vi "Devcon.Find Devices.vi"(8 "error in (no error)":errorcluster, 9 "State(Present(F), All(T))":bool, 10 "DeviceID":string="USB\\VID_28DE", 11 "DevconEXE":path=path "C:/Program Files (x86)/Windows Kits/10/Tools/x64/devcon") -> (0 "error out":errorcluster, 1 "StdOut":string, 2 "Device List":string[][](array[string]), 3 "Device Cnt":i32, 5 "Cmd":string)   [LabVIEW 2018]
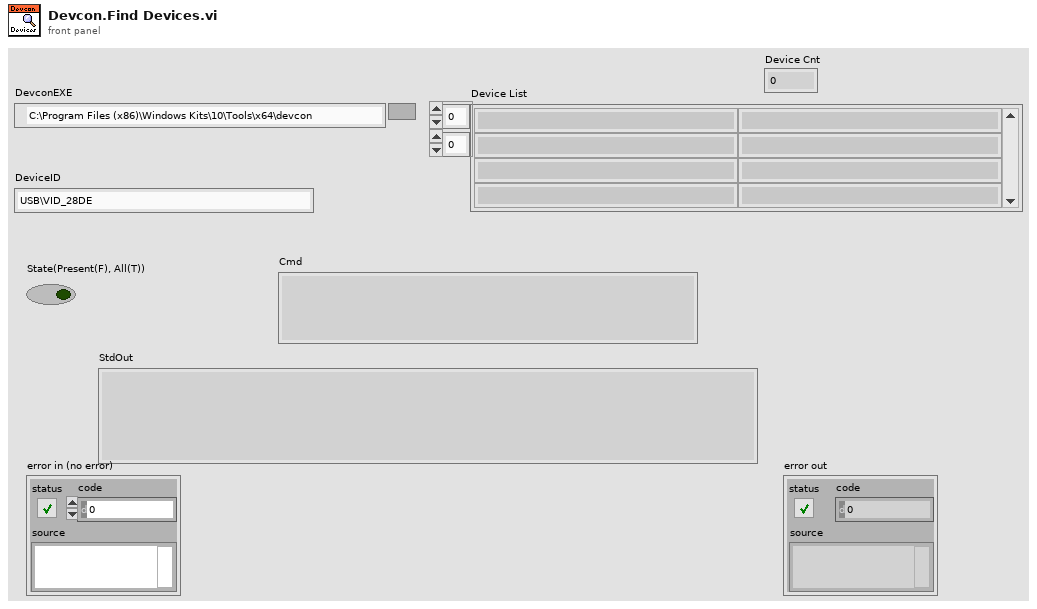
[diagram p1: front panel]
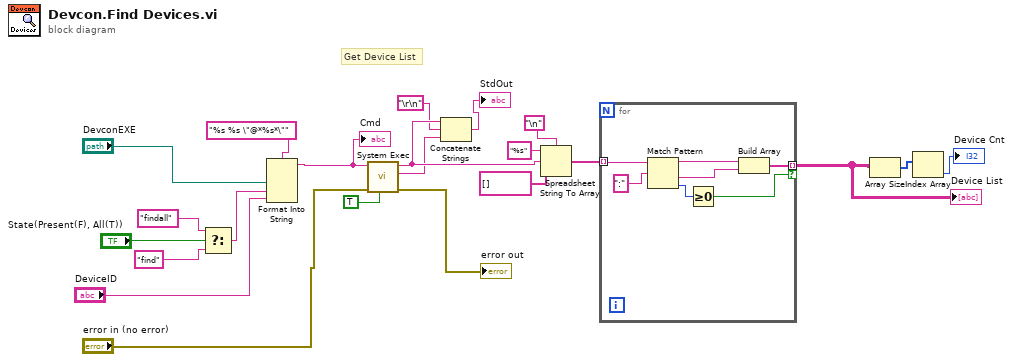
[diagram p0: block diagram]
diagram:
  # "Get Device List"
  n1 = Select(t="findall", s="State(Present(F), All(T))", f="find") -> (s? t:f=w5:string)
  n2 = Format Into String(format string="%s %s \"@*%s*\"", "DevconEXE", w5, "DeviceID") -> (resulting string=w19:string)  [unwired: 2 in, 1 out]
  "Cmd" <- w19
  n3 = call <vilib>:"System Exec.vi"("run minimized? (F)"=TRUE, "error in (no error)"="error in (no error)", "command line"=w19) -> ("error out"=→"error out":errorcluster, "standard error"=w3:string, "standard output"=w4:string)  [unwired: 5 in, 1 out]
  n4 = Concatenate Strings(w4, "\r\n", w3) -> (→"StdOut":string)
  n5 = Spreadsheet String To Array(delimiter (Tab)="\n", format string="%s", spreadsheet string=w4, array type (2D Dbl)=string[] [] ("Device List")) -> (array=w14:string[])
  n6 = for {
    tunnel: w14 -> [w29] mode=indexing
    tunnel: [w24] -> w13 mode=indexing if=w23
    n7 = Match Pattern(string=w29, regular expression=":") -> (before substring=w26:string, after substring=w25:string, offset past match=w27:i32)  [unwired: 1 in, 1 out]
    n8 = Greater Or Equal To 0?(x=w27) -> (x >= 0?=w23:bool)
    n9 = Build Array(w26, w25) -> (w24:string[])
  }
  "Device List" <- w13
  n10 = Array Size(array=w13) -> (size(s)=w12:i32[])
  n11 = Index Array(array=w12) -> (element=→"Device Cnt":i32)  [unwired: 1 in]
